vi "send_notification.vi"(0 "notification":i32, 1 "s":string) -> ()   [LabVIEW 2011]
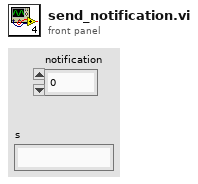
[diagram p1: front panel]
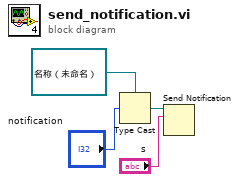
[diagram p0: block diagram]
diagram:
  n1 = Type Cast(type=refnum<notifier> refnum ("通知器输出"), x="notification") -> (*(type *) &x=w3:refnum<notifier>)
  n2 = Send Notification(notification="s", notifier=w3) -> ()  [unwired: 1 in, 2 out]
